vi "FlowRateSensorModel.vi"(10 "inputSignal(V)":dbl) -> (2 "FlowRate(LPM)":dbl)   [LabVIEW 2024]
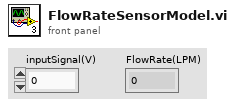
[diagram p1: front panel]
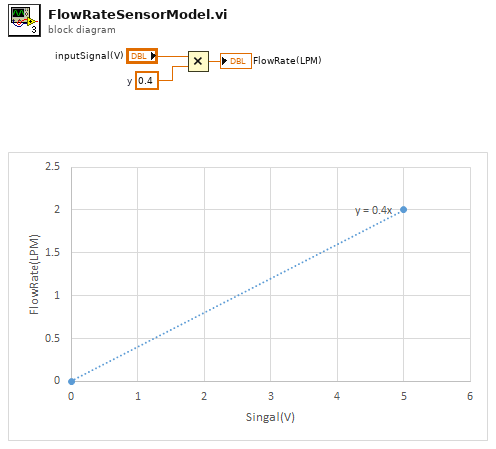
[diagram p0: block diagram]
diagram:
  w1 = 0.4  # y
  n1 = Multiply(x="inputSignal(V)", y=w1) -> (x*y=→"FlowRate(LPM)":dbl)
